vi "Close RFmx.vi"(8 "error in":errorcluster {"code" format="%.0x"}, 11 "Instrument Handle In":refnum<k21>) -> (0 "error out":errorcluster {"code" format="%.0x"})   [LabVIEW 2018]
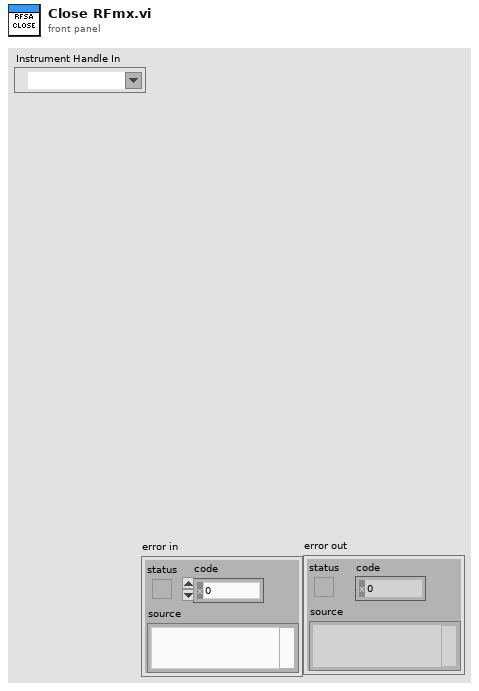
[diagram p1: front panel]
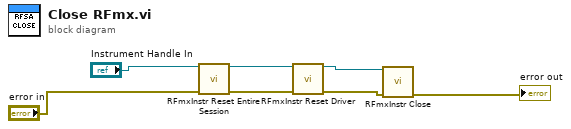
[diagram p0: block diagram]
diagram:
  n1 = call <vilib>:"RFmxInstr Reset Entire Session.vi"("Instrument Handle In"="Instrument Handle In", "error in (no error)"="error in") -> ("Instrument Handle Out"=w4:refnum<k21>, "error out"=w3:errorcluster)  [unwired: 12 in]
  n2 = call <vilib>:"RFmxInstr Reset Driver.vi"("Instrument Handle In"=w4, "error in (no error)"=w3) -> ("Instrument Handle Out"=w2:refnum<k21>, "error out"=w1:errorcluster)  [unwired: 12 in]
  n3 = call <vilib>:"RFmxInstr Close.vi"("Instrument Handle In"=w2, "error in (no error)"=w1) -> ("error out"=→"error out":errorcluster)  [unwired: 13 in]
